vi "Real QZ Decomposition.vi"(0 "A":T3, 5 "B":T3, 7 "decomposition type":i32(ring) items=["Generalized Hessenberg", "Generalized Schur"], 9 "order":T1 items=["No Reorder", "Real Ascending", "Real Descending", "Magnitude Ascending", "Magnitude Descending"]) -> (3 "Eigenvectors":T2, 4 "Q":T3, 6 "Z":T3, 8 "Alpha":cdb[](array[numeric]), 10 "Beta":dbl[](array[numeric]), 15 "error":i32)   [LabVIEW 2017, in "NI_AALPro.lvlib"]
doc: "Performs the QZ decomposition of a pair of square matrices. The data types you wire to the <B>A</B> and <B>B</B> inputs determine the polymorphic instance to use."
uses:
  NI_AALPro.lvlib
  RealMatrix.ctl
  ComplexMatrix.ctl
  Eigenvalue Order.ctl
  NI_Matrix.lvlib
  <resource>/lvanlys.dll
panel:
  # "QZ Decomposition"
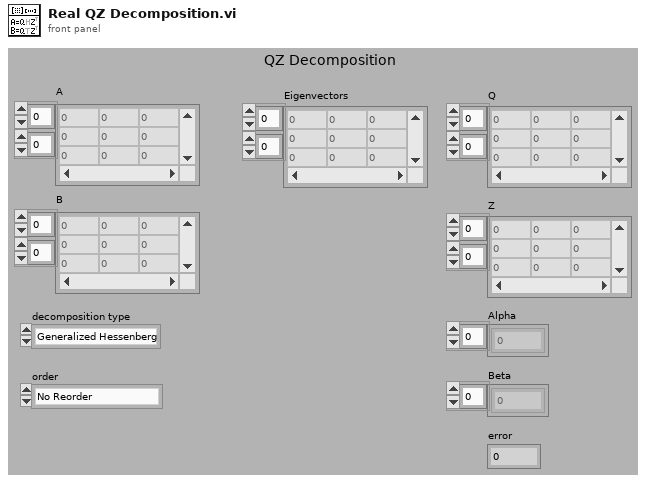
[diagram p1: front panel]
types:
  T1 = typedef "NI_AALPro.lvlib/Eigenvalue Order.ctl" = u16
  T2 = typedef "NI_Matrix.lvlib/ComplexMatrix.ctl" = cdb[][]
  T3 = typedef "NI_Matrix.lvlib/RealMatrix.ctl" = dbl[][]
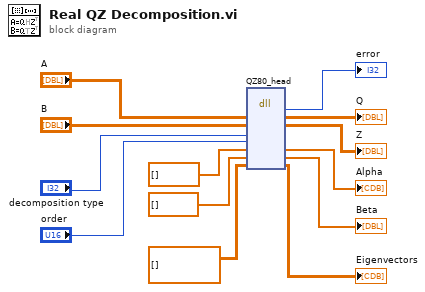
[diagram p0: block diagram]
diagram:
  n1 = dll-call lib="C:/Program Files (x86)/National Instruments/LabVIEW 2017/resource/lvanlys.*" fn="QZ80_head"("A"="A", "B"="B", "type"="decomposition type", "orderOpt"="order", "output param"=cdb[] [], "Beta"=dbl[] [], "Eigenvectors"=T2 []) -> (→"error":i32, "A"=→"Q":T3, "B"=→"Z":T3, "output param"=→"Alpha":cdb[], "Beta"=→"Beta":dbl[], "Eigenvectors"=→"Eigenvectors":T2)  [unwired: 5 in, 2 out]
